vi "numero primo.vi"() -> ()   [LabVIEW 2012]
panel:
  out "?":string
  in  "INGRESAR EL NUMERO":dbl
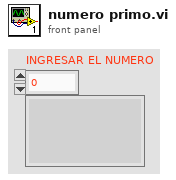
[diagram p1: front panel]
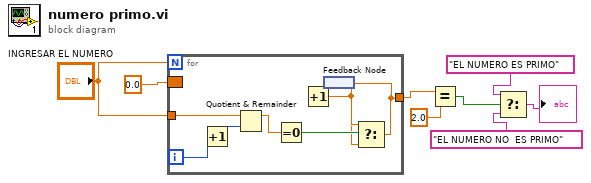
[diagram p0: block diagram]
diagram:
  n1 = for {
    N: "INGRESAR EL NUMERO" -> [_]
    tunnel: "INGRESAR EL NUMERO" -> [w15]
    tunnel: [w9] -> w7
    border: 0.0 -> [_]
    i -> [w16]
    n2 = Increment(x=w16) -> (x+1=w14:i32)
    n3 = Quotient & Remainder(x=w15, y=w14) -> (x-y*floor(x/y)=w13:dbl)  [unwired: 1 out]
    n4 = Equal To 0?(x=w13) -> (x = 0?=w12:bool)
    n5 = feedback #1() -> (w10:dbl)
    n6 = Increment(x=w10) -> (x+1=w11:dbl)
    n7 = Select(t=w11, s=w12, f=w10) -> (s? t:f=w9:dbl)
    n8 = feedback-in #1(w9) -> ()
  }
  n9 = Equal?(x=w7, y=2.0) -> (x = y?=w5:bool)
  n10 = Select(t="EL NUMERO ES PRIMO", s=w5, f="EL NUMERO NO  ES PRIMO") -> (s? t:f=→"?":string)
